vi "Load - Shoot - State Machine.vi"   [LabVIEW 2013]
uses:
  typedefs/singleUseSubstate.ctl
  typedefs/fg_typedef.ctl
  typedefs/subStates.ctl
types:
  T1 = typedef "singleUseSubstate.ctl" = enum16{"null", "wait", "shift high", "shift low", "extend shooter", "retract shooter", "close latch", "open latch"}
  T2 = typedef "subStates.ctl" = enum16{"null", "wait", "driver control", "auto", "manual override", "hold position", "rotate", "pickup", "pass", "load-shoot", "load-pass", "goto shoot", "shoot", "cancel", "end"}
  T3 = typedef "fg_typedef.ctl" = enum16{"Get", "Set"}
  T4 = typedef "WPI_DigitalInputDevRef.ctl" = cluster{"DevStatus":errorcluster, "DIO Channel":T5, "Digital Module":T6}
  T5 = typedef "FPGA_DIOChannel.ctl" = enum8{"DIO 1", "DIO 2", "DIO 3", "DIO 4", "DIO 5", "DIO 6", "DIO 7", "DIO 8", "DIO 9", "DIO 10", "DIO 11", "DIO 12", "DIO 13", "DIO 14", "Invalid"}
  T6 = typedef "FPGA_TypedefDigitalModule.ctl" = enum16{"Digital Module 1", "Digital Module 2"}
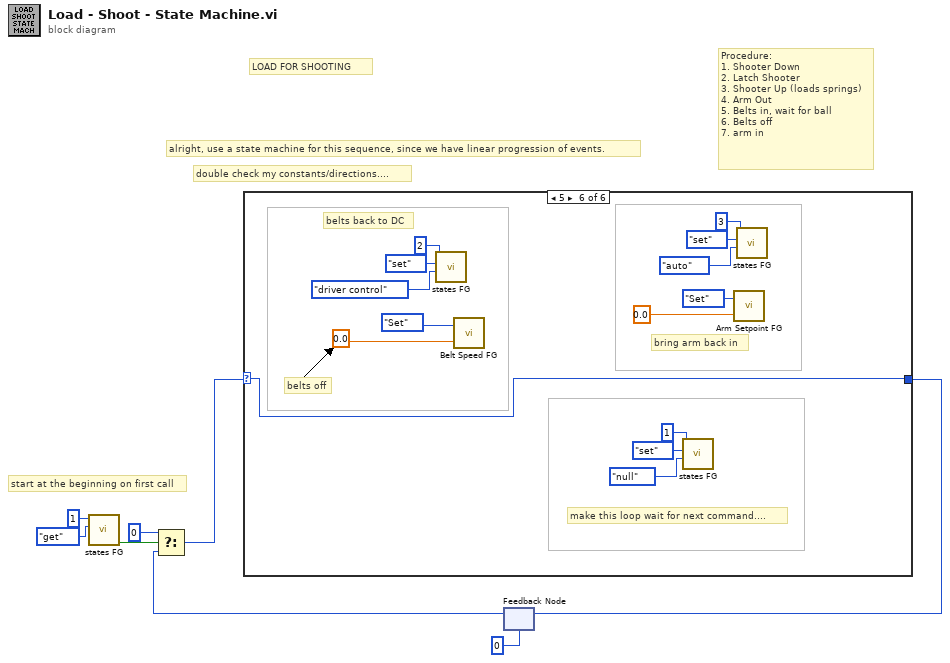
[diagram p0: block diagram]
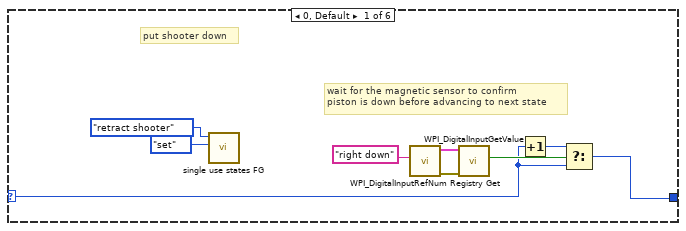
[diagram p2: hidden frame]
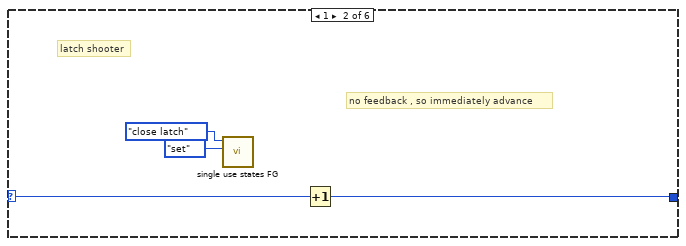
[diagram p3: hidden frame]
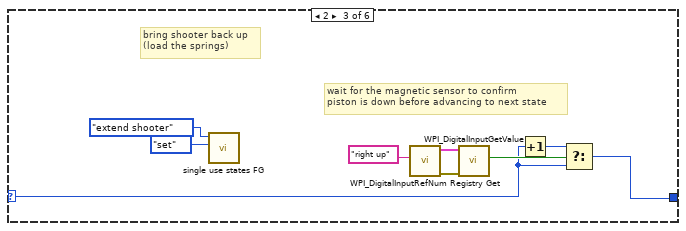
[diagram p4: hidden frame]
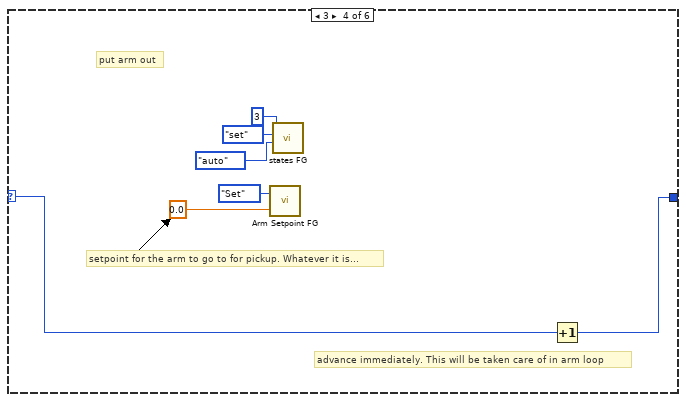
[diagram p5: hidden frame]
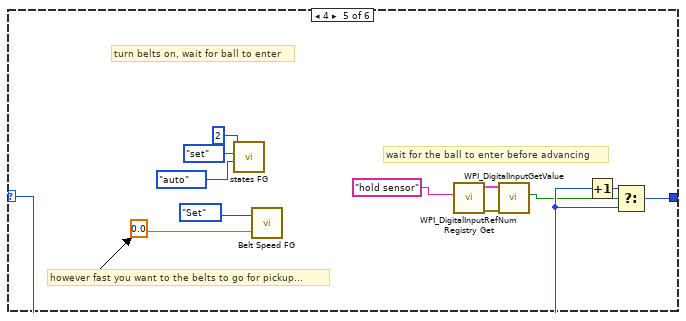
[diagram p6: hidden frame]
diagram:
  # "start at the beginning on first call"
  # "double check my constants/directions...."
  # "LOAD FOR SHOOTING"
  # "Procedure: \n1. Shooter Down\n2. Latch Shooter\n3. Shooter Up (loads springs)\n4. Arm Out\n5. Belts in, wait for ball\n6. Belts off\n7. arm in"
  # "alright, use a state machine for this sequence, since we have linear progression of events."
  n1 = call "states FG.vi"("menu (get)"=enum16{"set", "get"}."get", "Loop ID"=1) -> ("first call?"=w1:bool)  [unwired: 6 in, 3 out]
  n2 = feedback #1(0) -> (w4:i32)
  n3 = Select(t=0, s=w1, f=w4) -> (s? t:f=w3:i32)
  n4 = case shown="5" w3 {
    selector: w3 -> [w11 w21 w24 w32 w40 w50]
    tunnel: [w9 w18 w22 w31 w41 w50] -> w7
    frame 0, Default {
      # "wait for the magnetic sensor to confirm \npiston is down before advancing to next state"
      # "put shooter down"
      n5 = call "single use states FG.vi"("menu (get)"=enum16{"set", "get"}."set", "substate"=singleUseSubstate."retract shooter") -> ()  [unwired: 6 in, 4 out]
      n6 = call <vilib>:"WPI_DigitalInputRefNum Registry Get.vi"("refnum name"="right down") -> ("error out"=w14:errorcluster, "DigitalInputDevRef"=w13:T4)  [unwired: 9 in]
      n7 = call <vilib>:"WPI_DigitalInputGetValue.vi"("error in (no error)"=w14, "DigitalInputDevRef"=w13) -> ("Value"=w12:bool)  [unwired: 7 in, 2 out]
      n8 = Increment(x=w11) -> (x+1=w10:i32)
      n9 = Select(t=w10, s=w12, f=w11) -> (s? t:f=w9:i32)
    }
    frame 1 {
      # "no feedback , so immediately advance"
      # "latch shooter"
      n10 = call "single use states FG.vi"("menu (get)"=enum16{"set", "get"}."set", "substate"=singleUseSubstate."close latch") -> ()  [unwired: 6 in, 4 out]
      n11 = Increment(x=w21) -> (x+1=w18:i32)
    }
    frame 2 {
      # "wait for the magnetic sensor to confirm \npiston is down before advancing to next state"
      # "bring shooter back up\n(load the springs)"
      n12 = call "single use states FG.vi"("menu (get)"=enum16{"set", "get"}."set", "substate"=singleUseSubstate."extend shooter") -> ()  [unwired: 6 in, 4 out]
      n13 = call <vilib>:"WPI_DigitalInputRefNum Registry Get.vi"("refnum name"="right up") -> ("error out"=w27:errorcluster, "DigitalInputDevRef"=w26:T4)  [unwired: 9 in]
      n14 = call <vilib>:"WPI_DigitalInputGetValue.vi"("error in (no error)"=w27, "DigitalInputDevRef"=w26) -> ("Value"=w25:bool)  [unwired: 7 in, 2 out]
      n15 = Increment(x=w24) -> (x+1=w23:i32)
      n16 = Select(t=w23, s=w25, f=w24) -> (s? t:f=w22:i32)
    }
    frame 3 {
      # "advance immediately. This will be taken care of in arm loop"
      # "setpoint for the arm to go to for pickup. Whatever it is..."
      # "put arm out"
      n17 = call "Arm Setpoint FG.vi"("Setpoint In"=0.0, "Menu"=fg_typedef."Set") -> ()  [unwired: 1 out]
      n18 = call "states FG.vi"("subState in"=subStates."auto", "menu (get)"=enum16{"set", "get"}."set", "Loop ID"=3) -> ()  [unwired: 5 in, 4 out]
      n19 = Increment(x=w32) -> (x+1=w31:i32)
    }
    frame 4 {
      # "wait for the ball to enter before advancing"
      # "however fast you want to the belts to go for pickup..."
      # "turn belts on, wait for ball to enter"
      n20 = call "states FG.vi"("subState in"=subStates."auto", "menu (get)"=enum16{"set", "get"}."set", "Loop ID"=2) -> ()  [unwired: 5 in, 4 out]
      n21 = call "Belt Speed FG.vi"("Speed In"=0.0 ("Setpoint In"), "Menu"=fg_typedef."Set") -> ()  [unwired: 1 out]
      n22 = call <vilib>:"WPI_DigitalInputRefNum Registry Get.vi"("refnum name"="hold sensor") -> ("error out"=w43:errorcluster, "DigitalInputDevRef"=w42:T4)  [unwired: 9 in]
      n23 = call <vilib>:"WPI_DigitalInputGetValue.vi"("error in (no error)"=w43, "DigitalInputDevRef"=w42) -> ("Value"=w38:bool)  [unwired: 7 in, 2 out]
      n24 = Increment(x=w40) -> (x+1=w39:i32)
      n25 = Select(t=w39, s=w38, f=w40) -> (s? t:f=w41:i32)
    }
    frame 5 {
      # "make this loop wait for next command...."
      # "bring arm back in"
      # "belts back to DC"
      # "belts off"
      n26 = call "states FG.vi"("subState in"=subStates."driver control", "menu (get)"=enum16{"set", "get"}."set", "Loop ID"=2) -> ()  [unwired: 5 in, 4 out]
      n27 = call "Belt Speed FG.vi"("Speed In"=0.0 ("Setpoint In"), "Menu"=fg_typedef."Set") -> ()  [unwired: 1 out]
      n28 = call "states FG.vi"("subState in"=subStates."null", "menu (get)"=enum16{"set", "get"}."set", "Loop ID"=1) -> ()  [unwired: 5 in, 4 out]
      n29 = call "Arm Setpoint FG.vi"("Setpoint In"=0.0, "Menu"=fg_typedef."Set") -> ()  [unwired: 1 out]
      n30 = call "states FG.vi"("subState in"=subStates."auto", "menu (get)"=enum16{"set", "get"}."set", "Loop ID"=3) -> ()  [unwired: 5 in, 4 out]
    }
  }
  n31 = feedback-in #1(w7) -> ()
